vi "Bscan Script.vi"(7 "A-Scan Size":u32, 9 "Number of A-Scans":i32) -> (8 "spreadsheet string":string)   [LabVIEW 2012]
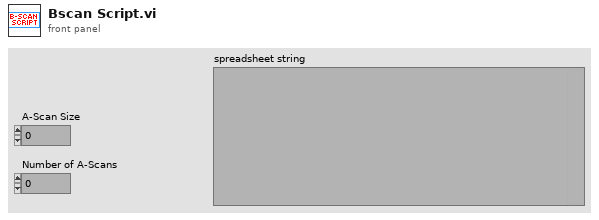
[diagram p1: front panel]
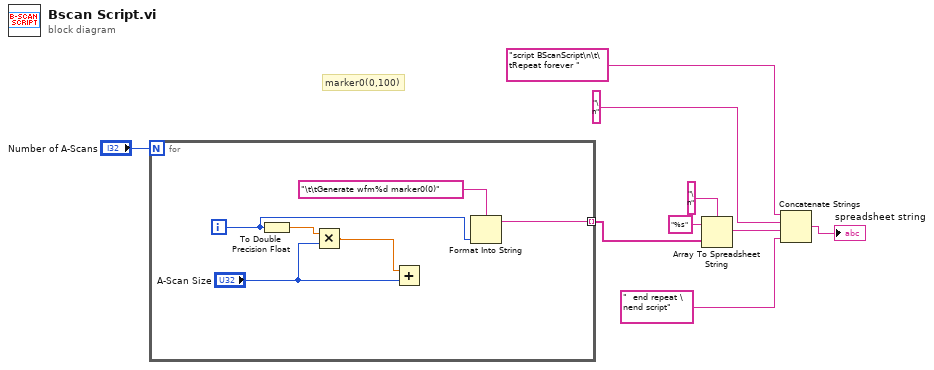
[diagram p0: block diagram]
diagram:
  # "marker0(0,100)"
  n1 = for {
    N: "Number of A-Scans" -> [_]
    tunnel: [w12] -> w8 mode=indexing
    i -> [w10]
    n2 = To Double Precision Float(number=w10) -> (double precision float=w13:dbl)
    n3 = Multiply(x=w13, y="A-Scan Size") -> (x*y=w11:dbl)
    n4 = Add(x=w11, y="A-Scan Size") -> ()  [unwired: 1 out]
    n5 = Format Into String(format string="\t\tGenerate wfm%d marker0(0)", w10) -> (resulting string=w12:string)  [unwired: 2 in, 1 out]
  }
  n6 = Array To Spreadsheet String(delimiter (Tab)="\n", array=w8, 3:"%s" ("format string")) -> (spreadsheet string=w4:string)
  n7 = Concatenate Strings("script BScanScript\n\t\tRepeat forever ", "\n" ("delimiter (Tab)"), w4, "  end repeat \nend script") -> (→"spreadsheet string":string)
